vi "Write to Port.vi"(10 "value":i16, 11 "AO in":refnum<class "AO0.lvclass">) -> ()   [LabVIEW 2017, in "Analog IO.lvlib" / "AO0.lvclass"]
uses:
  AO0.lvclass
  <vilib>/rvi/eio/common/nirviEmuTemplateMethod_errors.vi
  <vilib>/eio/EIONode/EIONode.xnode
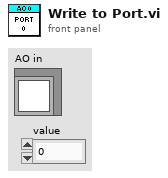
[diagram p1: front panel]
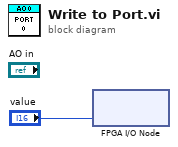
[diagram p0: block diagram]
diagram:
  n1 = xnode "FPGA I/O Node"("AO0"="value") -> ()  [unwired: 1 in, 1 out]
